vi "get initial information.vi"(8 "error in (no error)":errorcluster, 10 "SERN":u16, 11 "Simulated_CCD_Camera in":refnum<class "Sim_CCD.lvclass">) -> (0 "error out":errorcluster, 3 "Simulated_CCD_Camera out":refnum<class "Sim_CCD.lvclass">)   [LabVIEW 2018, in "Sim_CCD.lvclass"]
uses:
  Sim_CCD.lvclass
  Sim_CCD.lvclass/Sim_CCD.ctl
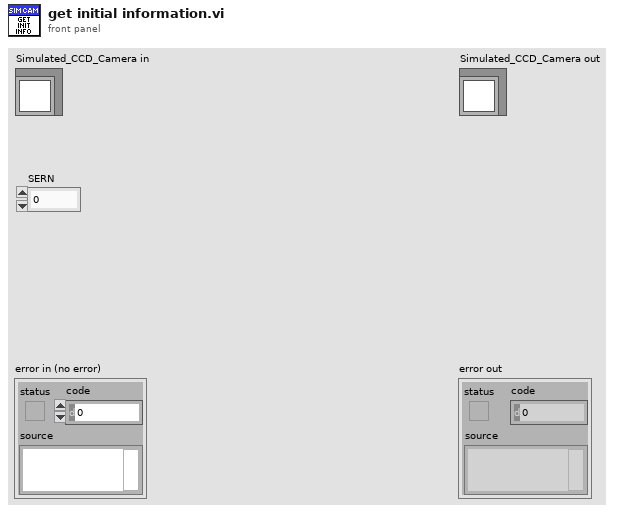
[diagram p1: front panel]
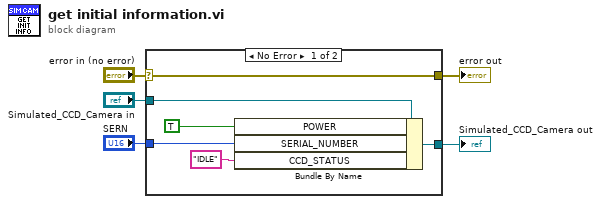
[diagram p0: block diagram]
diagram:
  n1 = case shown="No Error" "error in (no error)" {
    selector: "error in (no error)" -> [w11 w13]
    tunnel: [w11 w13] -> w3
    tunnel: [w7 w12] -> w2
    tunnel: "Simulated_CCD_Camera in" -> [w8 w12]
    tunnel: "SERN" -> [w6 _]
    frame No Error {
      n2 = Bundle By Name(cluster=w8, "POWER"=TRUE, "SERIAL_NUMBER"=w6, "CCD_STATUS"="IDLE" ("Camera Status.STATUS")) -> (w7:refnum<class "Sim_CCD.lvclass">)
    }
    frame Error {
    }
  }
  "error out" <- w3
  "Simulated_CCD_Camera out" <- w2
